vi "第1題.vi"() -> ()   [LabVIEW 2017]
uses:
  <vilib>/Utility/file.llb/Read Delimited Spreadsheet (DBL).vi
  <vilib>/Analysis/NI_AALBase.lvlib
panel:
  out "standard deviation(全部)":dbl format="%0.2f"
  out "mean2":dbl format="%0.2f"
  out "standard deviation(部分)":dbl format="%0.2f"
  out "mean":dbl format="%0.2f"
  out "取樣數":i32
  out "數據數":i32
  out "平均心跳":dbl
  out "熟睡心跳3點~7點":dbl
  out "熟睡時總心跳":dbl
  out "總心跳":dbl
  in  "file path (dialog if empty)":path
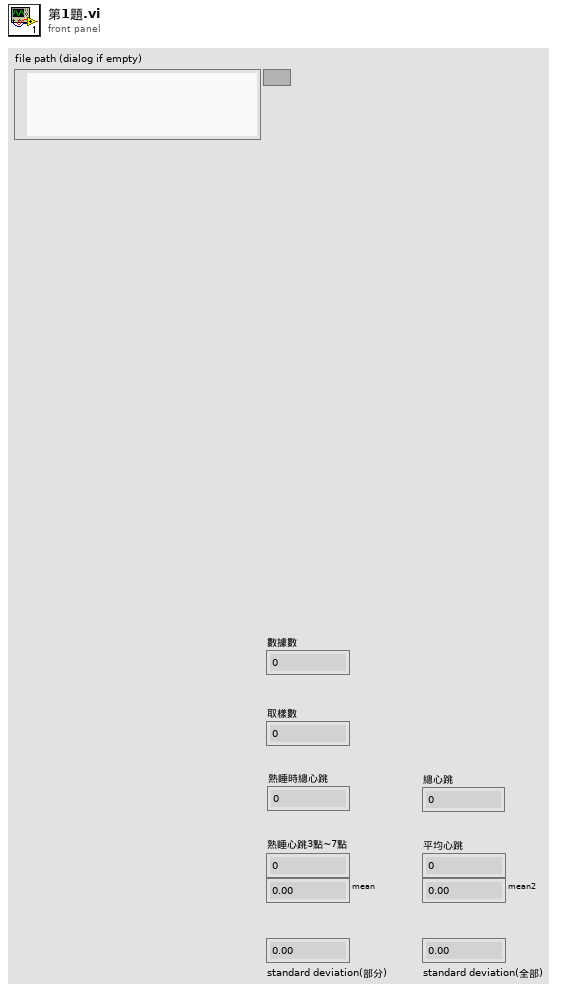
[diagram p1: front panel]
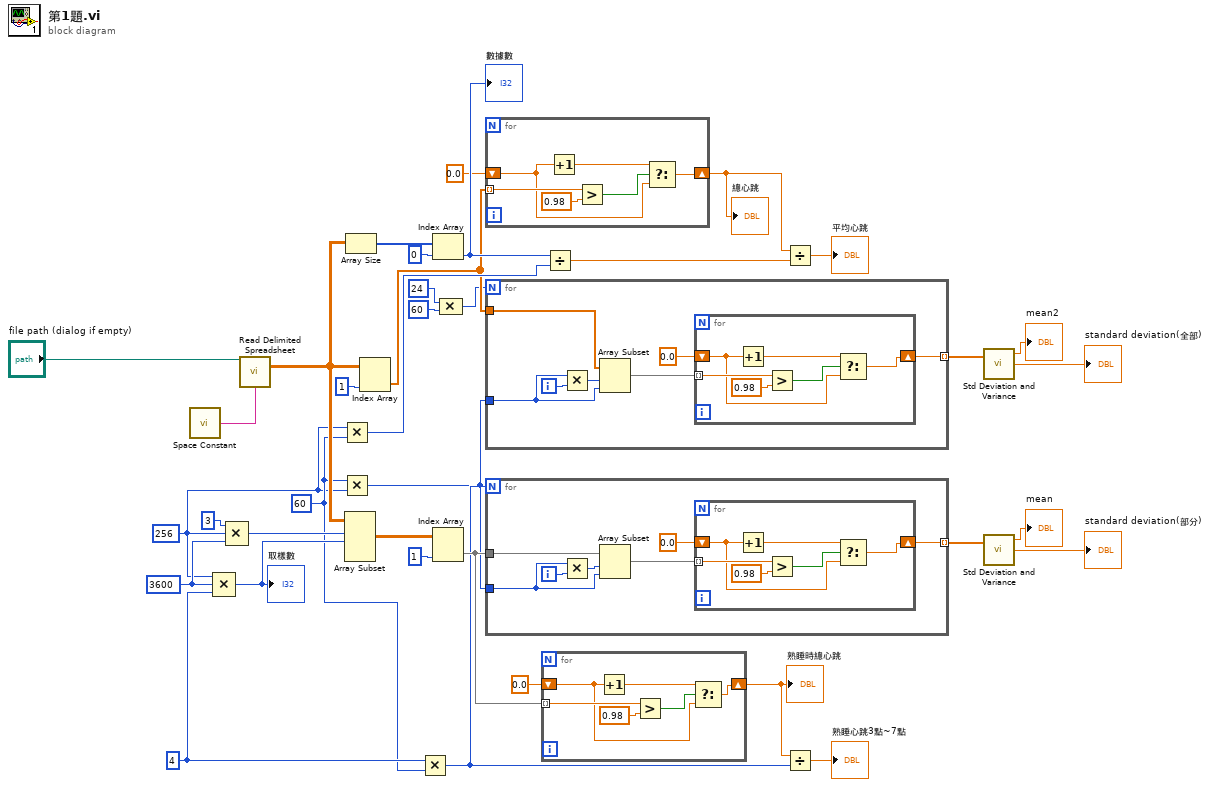
[diagram p0: block diagram]
diagram:
  w15 = 60
  w29 = 4
  w21 = 3600
  w14 = 256
  n1 = call <vilib>:"Space Constant.vi"() -> ("String"=w36:string)
  n2 = Compound Arithmetic op=MULTIPLY(w14, w21, w29) -> (w32:i32)
  "取樣數" <- w32
  n3 = Compound Arithmetic op=MULTIPLY(3, w14, w21) -> (w33:i32)
  n4 = call-poly <vilib>:"Read Delimited Spreadsheet.vi"("file path (dialog if empty)"="file path (dialog if empty)", "delimiter (\\t)"=w36) -> ("all rows"=w24:dbl[][])  [unwired: 8 in, 5 out]
  n5 = Multiply(x=w14, y=w15) -> (x*y=w20:i32)
  n6 = Multiply(x=w15, y=w14) -> (x*y=w6:i32)
  n7 = Array Subset(array=w24, index (row)=w33, length (row)=w32) -> (w30:dbl[][])  [unwired: 2 in]
  n8 = Array Size(array=w24) -> (size(s)=w23:i32[])
  n9 = Index Array(array=w24, index (col)=1) -> (element=w7:dbl[])  [unwired: 1 in]
  n10 = Multiply(x=w29, y=w15) -> (x*y=w16:i32)
  n11 = Index Array(array=w23, index=0) -> (element=w19:i32)
  "數據數" <- w19
  n12 = Index Array(array=w30, index (col)=1) -> (element=w17:dbl[])  [unwired: 1 in]
  n13 = Compound Arithmetic op=MULTIPLY(24, 60) -> (w3:i32)
  n14 = for {
    tunnel: w7 -> [w43] mode=indexing
    shift-right: [w40] -> w26
    shift-left: 0.0 -> [w38]
    n15 = Increment(x=w38) -> (x+1=w39:dbl)
    n16 = Greater?(x=w43, y=0.98) -> (0:w41:bool)
    n17 = Select(t=w39, s=w41, f=w38) -> (s? t:f=w40:dbl)
  }
  "總心跳" <- w26
  n18 = for {
    N: w3 -> [_]
    tunnel: w7 -> [w50]
    tunnel: w6 -> [w45]
    tunnel: [w46] -> w10 mode=indexing
    i -> [w49]
    n19 = Multiply(x=w45, y=w49) -> (x*y=w48:i32)
    n20 = Array Subset(array=w50, index=w48, length=w45) -> (w47:dbl[])
    n21 = for {
      tunnel: w47 -> [w56] mode=indexing
      shift-right: [w53] -> w46
      shift-left: 0.0 -> [w51]
      n22 = Increment(x=w51) -> (x+1=w52:dbl)
      n23 = Greater?(x=w56, y=0.98) -> (0:w54:bool)
      n24 = Select(t=w52, s=w54, f=w51) -> (s? t:f=w53:dbl)
    }
  }
  n25 = for {
    N: w16 -> [_]
    tunnel: w17 -> [w63]
    tunnel: w6 -> [w58]
    tunnel: [w59] -> w13 mode=indexing
    i -> [w62]
    n26 = Multiply(x=w58, y=w62) -> (x*y=w61:i32)
    n27 = Array Subset(array=w63, index=w61, length=w58) -> (w60:dbl[])
    n28 = for {
      tunnel: w60 -> [w69] mode=indexing
      shift-right: [w66] -> w59
      shift-left: 0.0 -> [w64]
      n29 = Increment(x=w64) -> (x+1=w65:dbl)
      n30 = Greater?(x=w69, y=0.98) -> (0:w67:bool)
      n31 = Select(t=w65, s=w67, f=w64) -> (s? t:f=w66:dbl)
    }
  }
  n32 = for {
    tunnel: w17 -> [w75] mode=indexing
    shift-right: [w72] -> w28
    shift-left: 0.0 -> [w70]
    n33 = Increment(x=w70) -> (x+1=w71:dbl)
    n34 = Greater?(x=w75, y=0.98) -> (0:w73:bool)
    n35 = Select(t=w71, s=w73, f=w70) -> (s? t:f=w72:dbl)
  }
  "熟睡時總心跳" <- w28
  n36 = Divide(x=w19, y=w20) -> (x/y=w18:dbl)
  n37 = Divide(x=w26, y=w18) -> (x/y=→"平均心跳":dbl)
  n38 = Divide(x=w28, y=w16) -> (x/y=→"熟睡心跳3點~7點":dbl)
  n39 = call <vilib>:"Std Deviation and Variance.vi"("X"=w10) -> ("mean"=→"mean2":dbl, "standard deviation"=→"standard deviation(全部)":dbl)  [unwired: 1 in, 1 out]
  n40 = call <vilib>:"Std Deviation and Variance.vi"("X"=w13) -> ("mean"=→"mean":dbl, "standard deviation"=→"standard deviation(部分)":dbl)  [unwired: 1 in, 1 out]
